vi "Set Version.vi"(8 "error in (no error)":errorcluster, 10 "Version":u8, 11 "UUID in":refnum<class "UUID.lvclass">) -> (0 "error out":errorcluster, 3 "UUID out":refnum<class "UUID.lvclass">)   [LabVIEW 2015, in "UUID.lvclass"]
uses:
  UUID.lvclass
  UUID.lvclass/UUID.ctl
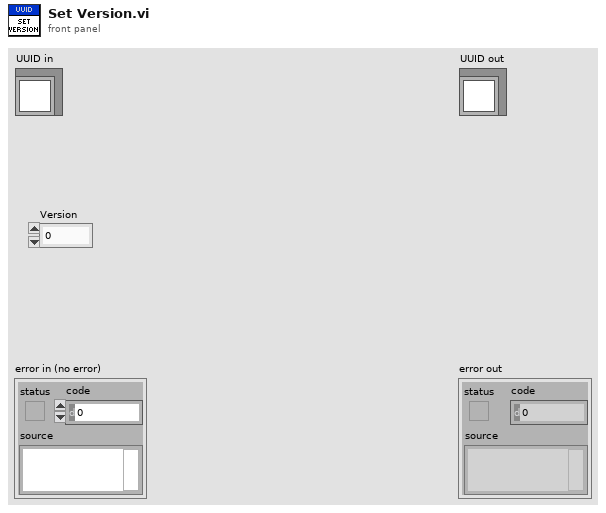
[diagram p1: front panel]
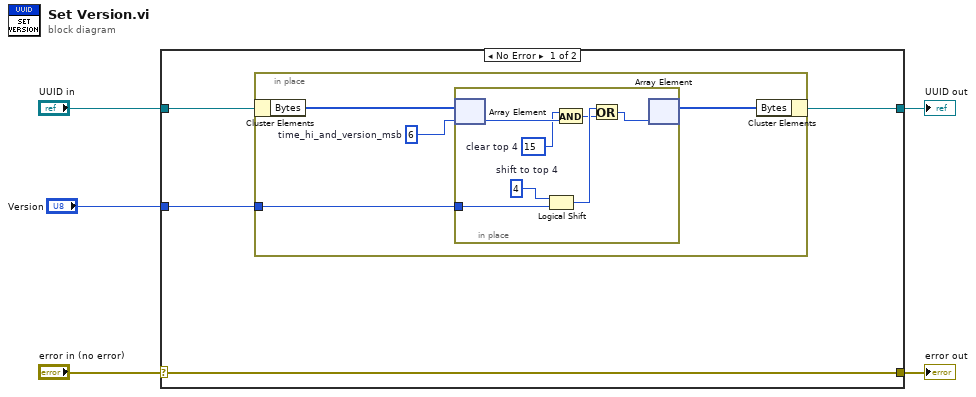
[diagram p0: block diagram]
diagram:
  n1 = case shown="No Error" "error in (no error)" {
    selector: "error in (no error)" -> [w9 w22]
    tunnel: [w9 w22] -> w4
    tunnel: [w7 w21] -> w2
    tunnel: "UUID in" -> [w8 w21]
    tunnel: "Version" -> [w6 _]
    frame No Error {
      n2 = in-place {
        in-place-border: w6 -> [w10]
        w11 = 6  # time_hi_and_version_msb
        n3 = in-place-cluster #1(w8) -> ("Bytes"=w13:u8[])
        n4 = in-place {
          in-place-border: w10 -> [w18]
          w14 = u8 15  # clear top 4
          w16 = i16 4  # shift to top 4
          n5 = in-place-array #2(w13, w11) -> (w20:u8)
          n6 = Logical Shift(y=w16, x=w18) -> (x << y=w17:u8)
          n7 = And(x=w14, y=w20) -> (x .and. y?=w15:u8)
          n8 = Or(x=w17, y=w15) -> (x .or. y?=w19:u8)
          n9 = in-place-array #2(w19) -> (w12:u8[])  [unwired: 1 out]
        }
        n10 = in-place-cluster #1("Bytes"=w12) -> (w7:refnum<class "UUID.lvclass">)
      }
    }
    frame Error {
    }
  }
  "error out" <- w4
  "UUID out" <- w2
